vi "Read String.vi"(8 "error in (no error)":errorcluster, 9 "Timeout (ms)":i32, 11 "CIFChannels in":refnum<class "CIFChannels.lvclass">) -> (0 "error out":errorcluster, 1 "timed out?":bool, 2 "Data":string, 3 "CIFChannels out":refnum<class "CIFChannels.lvclass">)   [LabVIEW 2021, in "CIFChannels.lvclass"]
uses:
  CIFChannels.lvclass
  ChannelCommon/typedef/Errors.ctl
  CIFChannels.lvclass/CIFChannels.ctl
  ChannelCommon/Utilities/Add Error Core.vi
  ChannelCommon/ChannelCommon.lvlib
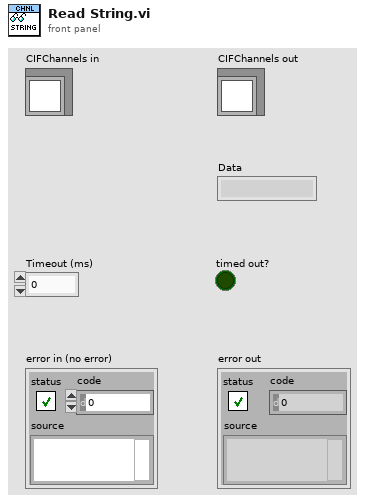
[diagram p1: front panel]
types:
  T1 = typedef "ChannelCommon.lvlib/Errors.ctl" = enum16{"gRPC Server Not Found", "Duplicate Channel", "Missing Channel", "Incorrect Type", "Flatten Error", "Unflatten Data", "Channel Length", "Plugin Connection", "gRPC Server Connection", "FIFO Unflatten", "Required Override", "Remove Not Found", "Multi Sub Not Supported", "Primary Already Connected", "Backpressure Not Supported", "Unable to Increase Buffer", "Data too Large"}
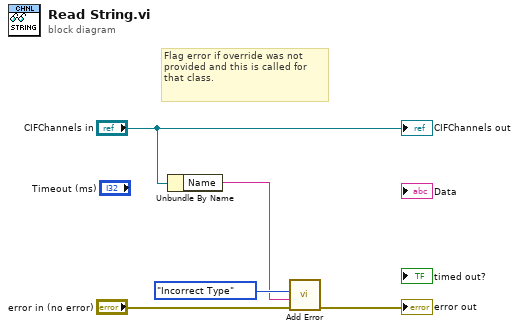
[diagram p0: block diagram]
diagram:
  # "Flag error if override was not provided and this is called for that class."
  n1 = Unbundle By Name("CIFChannels in") -> ("Name"=w1:string)
  n2 = call "Add Error.vi"("error in (no error)"="error in (no error)", "String to Append"=w1, "Error"=Errors."Incorrect Type") -> ("error out"=→"error out":errorcluster)  [unwired: 8 in]
  "CIFChannels out" <- "CIFChannels in"
